vi "Get All Instruments.vi"(8 "error in (no error)":errorcluster, 11 "ResourceEnumerator in":refnum<class "ResourceEnumerator.lvclass">) -> (0 "error out":errorcluster, 2 "Instruments":refnum<class "Driver.lvclass">[](array[class]), 3 "ResourceEnumerator out":refnum<class "ResourceEnumerator.lvclass">)   [LabVIEW 2023, in "HAF.lvlib" / "ResourceEnumerator.lvclass"]
doc: "Returns an array of Instrument Classes that are known to an application. They may or may not be connected to the System."
uses:
  ResourceEnumerator.lvclass
  ResourceEnumerator.lvclass/ResourceEnumerator.ctl
  DMM6500/DMM6500.lvclass
  HMC8043/HMC8043.lvclass
  SDS1104X-E/SDS1104X-E.lvclass
  Pico/Pico.lvclass
  SDG1032X/SDG1032X.lvclass
  ArduinoMega2560/ArduinoMega2560.lvclass
  ArduinoUnoR3/ArduinoUnoR3.lvclass
  Instrument Control Board/Instrument Control Board.lvclass
  \\Mac\Home/Documents/LabVIEW Data/ProjectTemplates/Source/HAF/SerialDriver/SerialDriver.lvclass
  \\Mac\Home/Documents/LabVIEW Data/ProjectTemplates/Source/HAF/Driver/Driver.lvclass
  \\Mac\Home/Documents/LabVIEW Data/ProjectTemplates/Source/HAF/Instrument Control Board/Instrument Control Board.lvclass
  \\Mac\Home/Documents/LabVIEW Data/ProjectTemplates/Source/HAF/ArduinoUnoR3/ArduinoUnoR3.lvclass
  \\Mac\Home/Documents/LabVIEW Data/ProjectTemplates/Source/HAF/ArduinoMega2560/ArduinoMega2560.lvclass
  \\Mac\Home/Documents/LabVIEW Data/ProjectTemplates/Source/HAF/Pico/Pico.lvclass
  \\Mac\Home/Documents/LabVIEW Data/ProjectTemplates/Source/HAF/SDG1032X/SDG1032X.lvclass
  \\Mac\Home/Documents/LabVIEW Data/ProjectTemplates/Source/HAF/SDS1104X-E/SDS1104X-E.lvclass
  \\Mac\Home/Documents/LabVIEW Data/ProjectTemplates/Source/HAF/HMC8043/HMC8043.lvclass
  \\Mac\Home/Documents/LabVIEW Data/ProjectTemplates/Source/HAF/DMM6500/DMM6500.lvclass
  Driver/Driver.lvclass
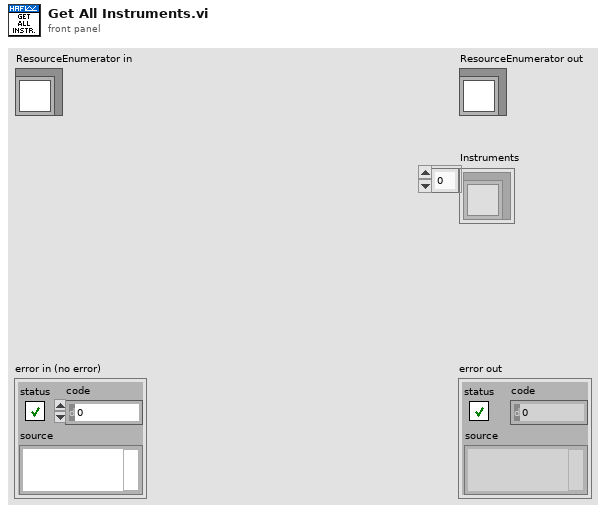
[diagram p1: front panel]
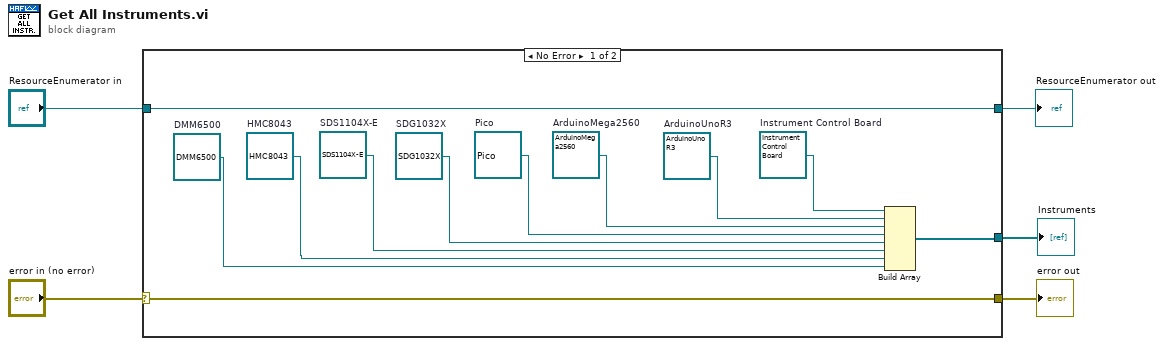
[diagram p0: block diagram]
diagram:
  n1 = case shown="No Error" "error in (no error)" {
    selector: "error in (no error)" -> [w15 w18]
    tunnel: [w15 w18] -> w3
    tunnel: [w16 w17] -> w1
    tunnel: "ResourceEnumerator in" -> [w16 w17]
    tunnel: [w8 _] -> w2
    frame No Error {
      w14 = refnum<class "Instrument Control Board.lvclass"> refnum  # Instrument Control Board
      w13 = refnum<class "ArduinoUnoR3.lvclass"> refnum  # ArduinoUnoR3
      w12 = refnum<class "ArduinoMega2560.lvclass"> refnum  # ArduinoMega2560
      w10 = refnum<class "SDG1032X.lvclass"> refnum  # SDG1032X
      w11 = refnum<class "Pico.lvclass"> refnum  # Pico
      w9 = refnum<class "SDS1104X-E.lvclass"> refnum  # SDS1104X-E
      w7 = refnum<class "HMC8043.lvclass"> refnum  # HMC8043
      w6 = refnum<class "DMM6500.lvclass"> refnum  # DMM6500
      n2 = Build Array(w14, w13, w12, w11, w10, w9, w7, w6) -> (w8:refnum<class "Driver.lvclass">[])
    }
    frame Error {
    }
  }
  "error out" <- w3
  "ResourceEnumerator out" <- w1
  "Instruments" <- w2
